vi "gaussmeter_test.vi"() -> ()   [LabVIEW 2016]
panel:
  out "name_1":string
  out "name_2":string
  out "name_3":string
  out "name_4":dbl
  out "test_result":dbl
  out "field":dbl
  out "error out":errorcluster
  in  "error in (no error)":errorcluster
  in  "VISA Resource Name":refnum<visa-resource-name>="Lakeshore_475"
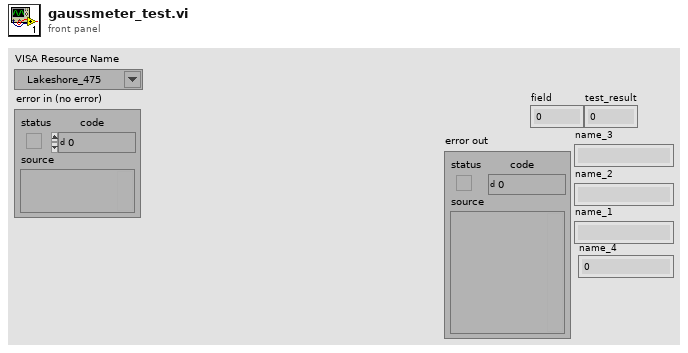
[diagram p1: front panel]
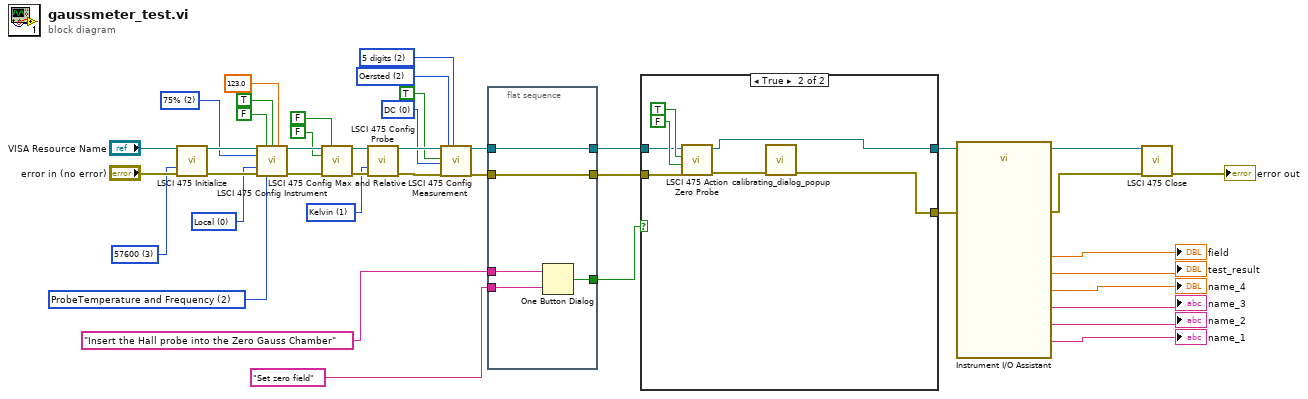
[diagram p0: block diagram]
diagram:
  w10 = u16 2 items=["3 digits", "4 digits", "5 digits"] ("DC Resolution (0: 3 digits)")
  w11 = u16 2 items=["Gauss", "Tesla", "Oersted", "Amp/meter"] ("Field Units (0: Gauss)")
  w12 = u16 0 items=["DC", "RMS", "Peak"] ("Measurement Mode (0: DC)")
  w16 = u16 1 items=["Celsius", "Kelvin"] ("Temperature Units (0: Celsius)")
  w23 = u16 2 items=["Blank", "Field", "ProbeTemperature and Frequency", "Relative Setpoint", "Field Control Setpoint", "Alarm Sort Message"] ("Display Line 2 (0: Blank)")
  w24 = u16 0 items=["Local", "Remote", "Remote with Local Lockout"] ("Remote Interface Mode (0: Local)")
  w25 = u16 2 items=["25%", "50%", "75%", "100%"] ("Display Brightness (0: 75%)")
  w40 = 3 items=["9600", "19200", "38400", "57600"] ("Baud Rate (0: 9600)")
  n1 = call <instrlib>:"LSCI 475 Initialize.vi"("VISA Resource Name"="VISA Resource Name", "Baud Rate (0: 9600)"=w40, "error in (no error)"="error in (no error)") -> ("VISA session"=w30:refnum<visa-resource-name>, "error out"=w29:errorcluster)  [unwired: 11 in]
  n2 = call <instrlib>:"LSCI 475 Config Instrument.vi"("VISA session"=w30, "Beep (F: Off)"=FALSE, "Keyboard Lock (F: Unlocked)"=TRUE, "Keyboard Lock Code (123)"=123.0, "Display Brightness (0: 75%)"=w25, "Remote Interface Mode (0: Local)"=w24, "error in (no error)"=w29, "Display Line 2 (0: Blank)"=w23) -> ("dup VISA session"=w22:refnum<visa-resource-name>, "error out"=w21:errorcluster)  [unwired: 6 in]
  n3 = call <instrlib>:"LSCI 475 Config Max and Relative.vi"("VISA session"=w22, "Relative Mode (F: Off)"=FALSE, "Max Hold (F: Off)"=FALSE, "error in (no error)"=w21) -> ("dup VISA session"=w18:refnum<visa-resource-name>, "error out"=w17:errorcluster)  [unwired: 10 in]
  n4 = call <instrlib>:"LSCI 475 Config Probe.vi"("VISA session"=w18, "Temperature Units (0: Celsius)"=w16, "error in (no error)"=w17) -> ("dup VISA session"=w15:refnum<visa-resource-name>, "error out"=w14:errorcluster)  [unwired: 11 in]
  n5 = call <instrlib>:"LSCI 475 Config Measurement.vi"("VISA session"=w15, "Auto Range (F: Off)"=TRUE, "Measurement Mode (0: DC)"=w12, "error in (no error)"=w14, "Field Units (0: Gauss)"=w11, "DC Resolution (0: 3 digits)"=w10) -> ("dup VISA session"=w7:refnum<visa-resource-name>, "error out"=w5:errorcluster)  [unwired: 12 in]
  n6 = flat-sequence {
    tunnel: w7 -> [w47]
    tunnel: [w47] -> w6
    tunnel: w5 -> [w46]
    tunnel: [w46] -> w4
    tunnel: "Set zero field" ("button name (\"OK\")") -> [w45]
    tunnel: "Insert the Hall probe into the Zero Gauss Chamber" ("message") -> [w44]
    tunnel: [w43] -> w1
    frame #0 {
      n7 = One Button Dialog(message=w44, button name ("OK")=w45) -> (true=w43:bool)
    }
  }
  n8 = case shown="True" w1 {
    tunnel: [w49 w50] -> w9
    tunnel: [w48 w51] -> w8
    tunnel: w6 -> [w49 w54]
    tunnel: w4 -> [w48 w53]
    frame False {
    }
    frame True {
      n9 = call <instrlib>:"LSCI 475 Action Zero Probe.vi"("error in (no error)"=w53, "Zero Probe (F: Do Not Zero)"=FALSE, "Clear Probe Zero  (F: Do Not Clear)"=TRUE, "VISA session"=w54) -> ("error out"=w52:errorcluster, "dup VISA session"=w50:refnum<visa-resource-name>)  [unwired: 6 in]
      n10 = call "calibrating_dialog_popup.vi"("error in (no error)"=w52) -> ("error out"=w51:errorcluster)  [unwired: 10 in]
    }
  }
  n11 = call "Instrument I/O Assistant"("Session In"=w9, "error in"=w8) -> ("Session Out"=w38:refnum<visa-resource-name>, "field"=→"field":dbl, "test_result"=→"test_result":dbl, "name_4"=→"name_4":dbl, "name_3"=→"name_3":string, "name_2"=→"name_2":string, "name_1"=→"name_1":string, "error out"=w37:errorcluster)  [unwired: 18 in]
  n12 = call <instrlib>:"LSCI 475 Close.vi"("VISA session"=w38, "error in (no error)"=w37) -> ("error out"=→"error out":errorcluster)  [unwired: 13 in]
